vi "INI_Dialog display options_Cluster.vi"(7 "File Action":enum16{"Read", "Write"}(ring), 8 "error in (no error)":errorcluster, 11 "Hide Full Names":bool) -> (0 "error out":errorcluster, 3 "Hide Full Names Out":bool)   [LabVIEW 2023]
uses:
  <vilib>/Utility/config.llb/NI_LVConfig.lvlib
  <userlib>/_OpenG.lib/variantconfig/variantconfig.llb/openg_variant_configuration_file.lvlib
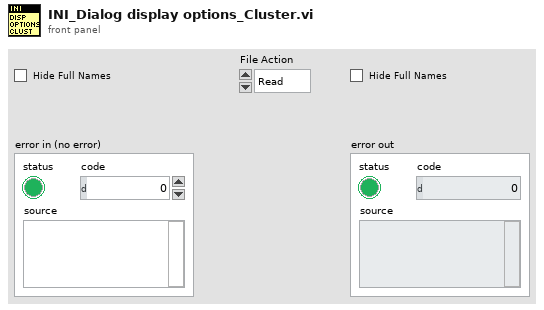
[diagram p1: front panel]
types:
  T1 = typedef "NI_LVConfig.lvlib/Config Data RefNum.ctl" = refnum<k1>
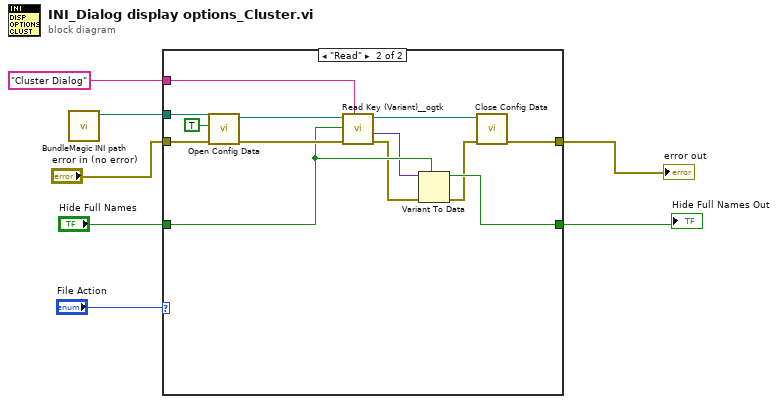
[diagram p0: block diagram]
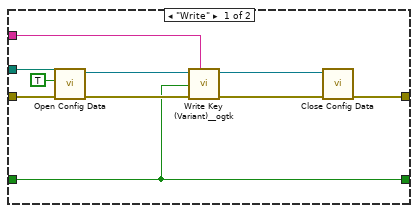
[diagram p2: hidden frame]
diagram:
  n1 = call "BundleMagic INI path.vi"() -> ("appended path"=w4:path)  [unwired: 11 in]
  n2 = case shown="\"Read\"" "File Action" {
    tunnel: w4 -> [w13 w27]
    tunnel: "Hide Full Names" -> [w11 w25]
    tunnel: [w11 w23] -> w5
    tunnel: "error in (no error)" -> [w10 w22]
    tunnel: [w9 w21] -> w2
    tunnel: "Cluster Dialog" ("section") -> [w8 w18]
    frame "Write" {
      n3 = call <vilib>:"Open Config Data.vi"("error in (no error)"=w10, "create file if necessary (T)"=TRUE, "configuration file path"=w13) -> ("error out"=w15:errorcluster, "refnum"=w17:T1)  [unwired: 6 in, 1 out]
      n4 = call <userlib>:"Write Key (Variant)__ogtk.vi"("section"=w8, "error in (no error)"=w15, "key-value"=w11, "refnum"=w17) -> ("error out"=w14:errorcluster, "refnum out"=w16:T1)  [unwired: 6 in]
      n5 = call <vilib>:"Close Config Data.vi"("error in (no error)"=w14, "refnum"=w16) -> ("error out"=w9:errorcluster)  [unwired: 8 in, 1 out]
    }
    frame "Read" {
      n6 = call <vilib>:"Open Config Data.vi"("error in (no error)"=w22, "create file if necessary (T)"=TRUE, "configuration file path"=w27) -> ("error out"=w28:errorcluster, "refnum"=w30:T1)  [unwired: 6 in, 1 out]
      n7 = call <userlib>:"Read Key (Variant)__ogtk.vi"("section"=w18, "error in (no error)"=w28, "type"=w25, "refnum"=w30) -> ("error out"=w20:errorcluster, "key-value"=w24:variant, "refnum out"=w29:T1)  [unwired: 4 in, 1 out]
      n8 = Variant To Data(error in=w20, type=w25, Variant=w24) -> (data=w23:bool, error out=w19:errorcluster)
      n9 = call <vilib>:"Close Config Data.vi"("error in (no error)"=w19, "refnum"=w29) -> ("error out"=w21:errorcluster)  [unwired: 8 in, 1 out]
    }
  }
  "Hide Full Names Out" <- w5
  "error out" <- w2
